vi "OC2 Setup Control.vi"(3 "error in (no error)":errorcluster, 4 "control type report in":T1 {"Power up state" items=["Off", "On", "Last"]; "Dead Band" format="%.2f"; "Derivative TC" format="%.1f"; "Derivative" format="%.2f"; "Integral" format="%.1f"; "Proportional Gain" format="%.1f"; "Control Type" items=["Off", "On/Off", "P", "PI", "PID"]}, 5 "enable":bool, 6 "VISA resource name":refnum<visa-resource-name>) -> (0 "error out":errorcluster, 1 "control type report out":T1 {"Power up state" items=["Off", "On", "Last"]; "Dead Band" format="%.2f"; "Derivative TC" format="%.1f"; "Derivative" format="%.2f"; "Integral" format="%.1f"; "Proportional Gain" format="%.1f"; "Control Type" items=["Off", "On/Off", "P", "PI", "PID"]}, 2 "dup VISA resource name":refnum<visa-resource-name>)   [LabVIEW 2009]
doc: "TCM Setup Control.vi\n\nVI that sets the control information, accepts a cluster that contains the following variables:\nControl Type - off, PID etc\nProportional gain - control proportional gain (P term)\nIntergral - control integral (i term)\nDerivative - control derivative (D term)\nDerivative TC\nDead Band\nPower up state - off the control is not on when tcm starts, on control is on with tcm power up\n\nCOPYRIGHT ELECTRON DYNAMICS LTD"
panel:
  out "write data":string
  # "Setup control variables"
  # "V1.02"
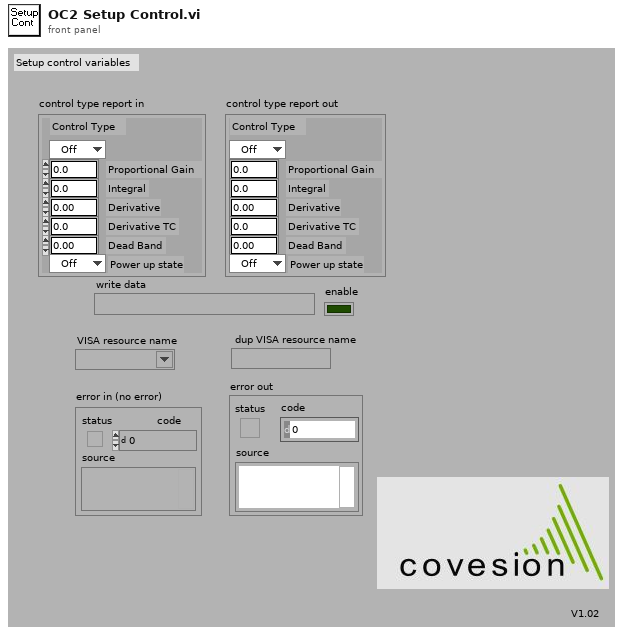
[diagram p1: front panel]
types:
  T1 = cluster{"Control Type":u16, "Proportional Gain":dbl, "Integral":dbl, "Derivative":dbl, "Derivative TC":dbl, "Dead Band":dbl, "Power up state ":u16}
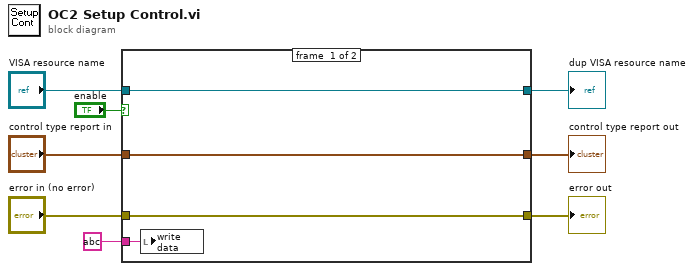
[diagram p0: block diagram]
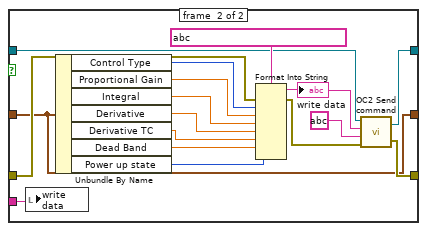
[diagram p2: hidden frame]
diagram:
  n1 = case shown="True" "enable" {
    tunnel: "control type report in" -> [w10 w15]
    tunnel: "VISA resource name" -> [w12 w19]
    tunnel: "error in (no error)" -> [w11 w18]
    tunnel: [w11 w16] -> w5
    tunnel: [w12 w14] -> w4
    tunnel: [w10 w15] -> w3
    tunnel: string ? ("write data") -> [w9 w13]
    frame #0 {
      n2 = local write "write data"(w9) -> ()
    }
    frame #1 {
      n3 = local write "write data"(w13) -> ()
      n4 = Unbundle By Name(w15) -> ("Control Type"=w20:u16, "Proportional Gain"=w21:dbl, "Integral"=w22:dbl, "Derivative"=w23:dbl, "Derivative TC"=w24:dbl, "Dead Band"=w25:dbl, "Power up state"=w26:u16)
      n5 = Format Into String(format string=string ?, error in=w18, w20, w21, w22, w23, w24, w25, w26) -> (resulting string=w27:string, error out=w17:errorcluster)  [unwired: 1 in]
      "write data" <- w27
      n6 = call "OC2 Send command.vi"("VISA resource name"=w19, "Command data"=w27, "Command"=string ?, "error in (no error)"=w17) -> ("dup VISA resource name"=w14:refnum<visa-resource-name>, "error out"=w16:errorcluster)  [unwired: 1 in]
    }
  }
  "dup VISA resource name" <- w4
  "error out" <- w5
  "control type report out" <- w3
